vi "Configure Arbitrary Waveform.vi"(0 "VISA resource name":refnum<visa-resource-name>, 1 "Waveform File Is Specified (F: No)":bool, 2 "Amplitude (0.1 Vpp)":dbl=0.1, 5 "Channel (1: 1)":i32(ring)=1 items=["1"=1, "2"=2], 7 "Sample Rate (40000 Sa/s)":dbl=40000.0, 9 "Offset (0 V)":dbl, 11 "error in (no error)":errorcluster, 12 "Arbitrary Waveform (ARB1)":string="ARB1", 13 "Amplitude Unit (0: Vpp)":u16(ring) items=["Vpp", "VRMS", "DBM"]) -> (4 "VISA resource name out":refnum<visa-resource-name>, 15 "error out":errorcluster)   [LabVIEW 2013, in "AWG.lvlib" / "Agilent 3352X Series.lvlib"]
doc: "Select an arbitrary waveform segment or sequence in volatile memory or non-volatile storage(.arb, .barb or .seq File), sets the waveform parameters and make it the active waveform function. \n\n<b>Note</b>: \nThe amplitude and offset value pair is restricted by voltage limit. Use Configure voltage limits.vi to adjust voltage limit if you really want."
uses:
  Agilent 3352X Series.lvlib
panel:
  # "Amplitude Settings"
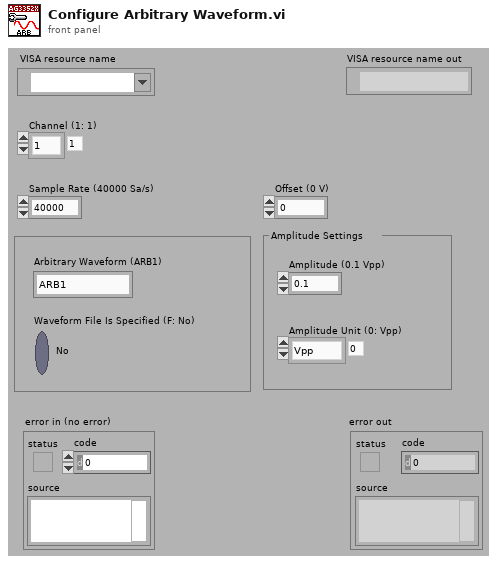
[diagram p1: front panel]
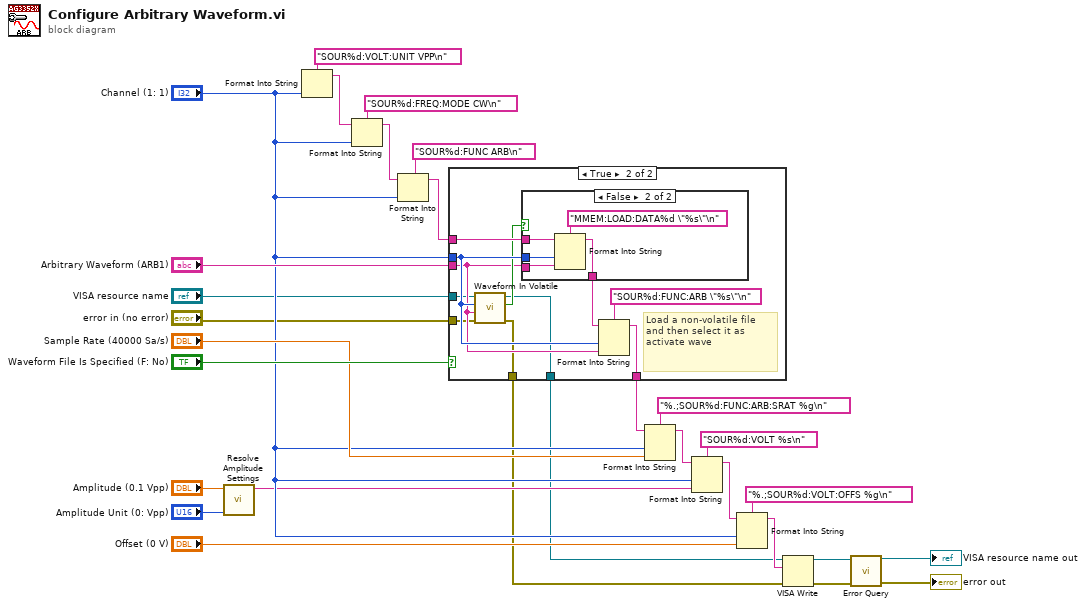
[diagram p0: block diagram]
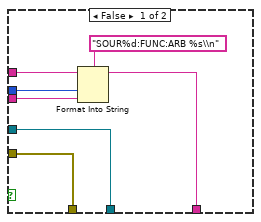
[diagram p2: hidden frame]
diagram:
  n1 = call "Resolve Amplitude Settings.vi"("Amplitude Unit (0: VPP)"="Amplitude Unit (0: Vpp)", "Amplitude (1 Vpp)"="Amplitude (0.1 Vpp)") -> ("Resulting String"=w9:string)  [unwired: 9 out]
  n2 = Format Into String(format string="SOUR%d:VOLT:UNIT VPP\n", "Channel (1: 1)") -> (resulting string=w15:string)  [unwired: 2 in, 1 out]
  n3 = Format Into String(format string="SOUR%d:FREQ:MODE CW\n", initial string=w15, "Channel (1: 1)") -> (resulting string=w17:string)  [unwired: 1 in, 1 out]
  n4 = Format Into String(format string="SOUR%d:FUNC ARB\n", initial string=w17, "Channel (1: 1)") -> (resulting string=w19:string)  [unwired: 1 in, 1 out]
  n5 = case shown="True" "Waveform File Is Specified (F: No)" {
    tunnel: "Channel (1: 1)" -> [w33 w43]
    tunnel: "Arbitrary Waveform (ARB1)" -> [w32 w41]
    tunnel: w19 -> [w35 w47]
    tunnel: [w34 w44] -> w16
    tunnel: "VISA resource name" -> [w30 w40]
    tunnel: "error in (no error)" -> [w31 w39]
    tunnel: [w30 w38] -> w2
    tunnel: [w31 w37] -> w1
    frame False {
      n6 = Format Into String(format string="SOUR%d:FUNC:ARB %s\\n", initial string=w35, w33, w32) -> (resulting string=w34:string)  [unwired: 1 in, 1 out]
    }
    frame True {
      # "Load a non-volatile file and then select it as activate wave"
      n7 = call "Waveform In Volatile.vi"("error in (no error)"=w39, "Arbitrary Waveform Name"=w41, "Channel (1: 1)"=w43, "VISA resource name"=w40) -> ("error out"=w37:errorcluster, "Wave In Volatile?"=w42:bool, "VISA resource name out"=w38:refnum<visa-resource-name>)  [unwired: 5 out]
      n8 = case shown="False" w42 {
        tunnel: w47 -> [w48 w52]
        tunnel: [w48 w51] -> w45
        tunnel: w41 -> [_ w50]
        tunnel: w43 -> [_ w49]
        frame True {
          # "Skip loading if waveform already in volatile memory"
        }
        frame False {
          n9 = Format Into String(format string="MMEM:LOAD:DATA%d \"%s\"\n", initial string=w52, w49, w50) -> (resulting string=w51:string)  [unwired: 1 in, 1 out]
        }
      }
      n10 = Format Into String(format string="SOUR%d:FUNC:ARB \"%s\"\n", initial string=w45, w43, w41) -> (resulting string=w44:string)  [unwired: 1 in, 1 out]
    }
  }
  n11 = Format Into String(format string="%.;SOUR%d:FUNC:ARB:SRAT %g\n", initial string=w16, "Channel (1: 1)", "Sample Rate (40000 Sa/s)") -> (resulting string=w13:string)  [unwired: 1 in, 1 out]
  n12 = Format Into String(format string="SOUR%d:VOLT %s\n", initial string=w13, "Channel (1: 1)", w9) -> (resulting string=w11:string)  [unwired: 1 in, 1 out]
  n13 = Format Into String(format string="%.;SOUR%d:VOLT:OFFS %g\n", initial string=w11, "Channel (1: 1)", "Offset (0 V)") -> (resulting string=w10:string)  [unwired: 1 in, 1 out]
  n14 = VISA Write(VISA resource name=w2, write buffer=w10, error in (no error)=w1) -> (VISA resource name out=w6:refnum<visa-resource-name>, error out=w5:errorcluster)  [unwired: 1 out]
  n15 = call "Error Query.vi"("error in (no error)"=w5, "VISA resource name"=w6) -> ("error out"=→"error out":errorcluster, "VISA resource name out"=→"VISA resource name out":refnum<visa-resource-name>)  [unwired: 8 out]
